vi "Add Terminals to Connector Pane.vi"() -> ()   [LabVIEW 2019]
doc: "Run this VI to assign the controls and indicators of Test - Connector Pane.vi to terminals in the specified connector pane pattern.\n\nFor a list of valid connector pane pattern values, see the Connector Pane Pattern Reference.vi.\n\nThe Detailed Help explains how this example illustrates a general procedure for assigning front panel controls and indicators to a connector pane programmatically."
panel:
  in  "vi path":path=path "Test - Connector Pane.vi"
  in  "Connector Pane Pattern":u32=4814
  # "Select Help>>Show Context Help and move the cursor over the VI icon to display help for this VI.\n\nBefore you start: Open the Detailed Help for this example to display the Configuring a Connector Pane Using VI Scripting topic in the  LabVIEW Help. That topic provides additional details about how this example illustrates the general procedure for assigning front panel controls and indicators to a connector pane programmatically."
  # "Overview: Demonstrates the use of VI Scripting to programmatically assign controls and indicators to a VI's connector pane.\nInstructions:\n1. Open Test - Connector Pane.vi.\n2. Run this VI. Observe the changes to the connector pane of the Test VI."
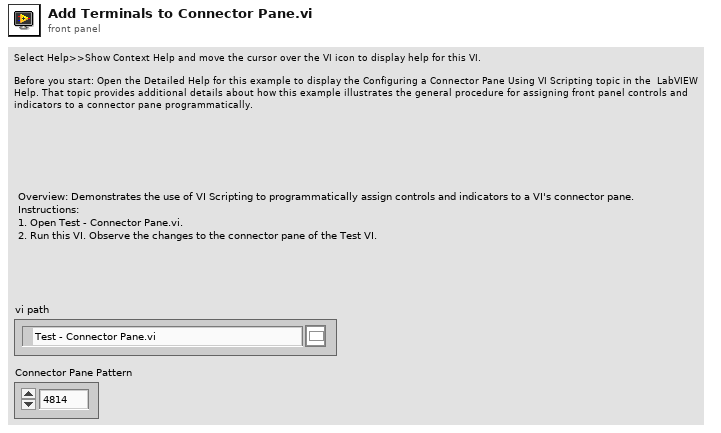
[diagram p1: front panel]
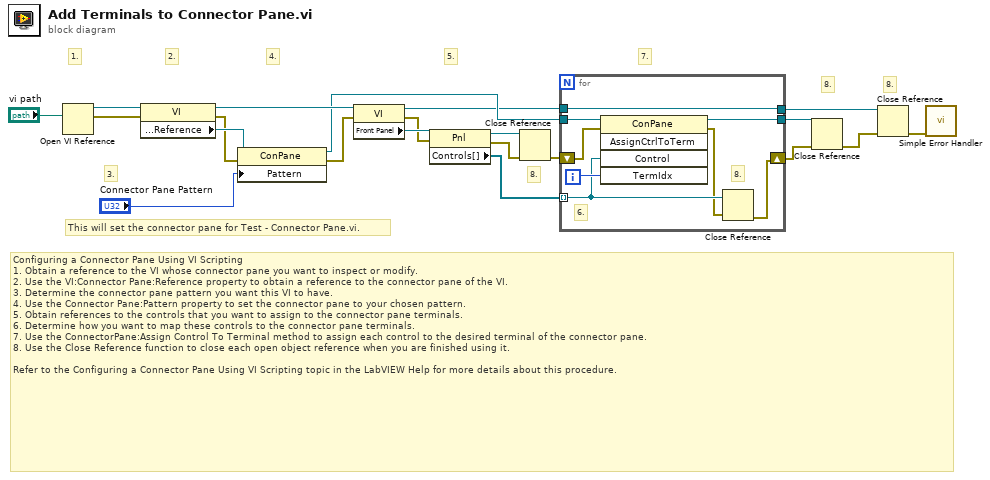
[diagram p0: block diagram]
diagram:
  # "8."
  # "8."
  # "8."
  # "7."
  # "3."
  # "5."
  # "4."
  # "2."
  # "1."
  # "Configuring a Connector Pane Using VI Scripting\n1. Obtain a reference to the VI whose connector pane you want to inspect or modify.\n2. Use the VI:Connector Pane:Reference property to obtain a reference to the connector pane of the VI.\n3. Determine the connector pane pattern you want this VI to have.\n4. Use the Connector Pane:Pattern property to set the connector pane to your chosen pattern.\n5. Obtain references to the controls that you want to assign to the connector pane terminals.\n6. Determine how you want to map these controls to the connector pane terminals.\n7. Use the ConnectorPane:Assign Control To Terminal method to assign each control to the desired terminal of the connector pane.\n8. Use the Close Reference function to close each open object reference when you are finished using it.\n\nRefer to the Configuring a Connector Pane Using VI Scripting topic in the LabVIEW Help for more details about this procedure."
  # "This will set the connector pane for Test - Connector Pane.vi."
  n1 = Open VI Reference(vi path="vi path") -> (vi reference=w2:refnum<vi>, error out=w3:errorcluster)  [unwired: 2 in, 3 out]
  n2 = property class="VI"(reference=w2, error in=w3) -> (reference out=w21:refnum<vi>, error out=w15:errorcluster, "Connector Pane:Reference"=w17:refnum<vi>)
  n3 = property class="ConPane"(reference=w17, error in=w15, "Pattern"="Connector Pane Pattern") -> (reference out=w14:refnum<vi>, error out=w16:errorcluster)
  n4 = property class="VI"(reference=w21, error in=w16) -> (reference out=w13:refnum<vi>, error out=w19:errorcluster, "Front Panel"=w20:refnum<vi>)
  n5 = property class="Pnl"(reference=w20, error in=w19) -> (reference out=w12:refnum<vi>, error out=w11:errorcluster, "Controls[]"=w18:refnum<vi>[])
  n6 = Close Reference(reference=w12, error in (no error)=w11) -> (error out=w10:errorcluster)
  n7 = for {
    tunnel: w18 -> [w24] mode=indexing
    tunnel: w14 -> [w29]
    shift-right: [w25] -> w8
    shift-left: w10 -> [w28]
    tunnel: [w26] -> w6
    tunnel: w13 -> [w26]
    tunnel: [w22] -> w7
    i -> [w27]
    # "8."
    # "6."
    n8 = invoke class="ConPane" method="AssignCtrlToTerm"(reference=w29, error in=w28, "Control"=w24, "TermIdx"=w27) -> (reference out=w22:refnum<vi>, error out=w23:errorcluster)  [unwired: 1 in, 3 out]
    n9 = Close Reference(reference=w24, error in (no error)=w23) -> (error out=w25:errorcluster)
  }
  n10 = Close Reference(reference=w7, error in (no error)=w8) -> (error out=w5:errorcluster)
  n11 = Close Reference(reference=w6, error in (no error)=w5) -> (error out=w1:errorcluster)
  n12 = call <vilib>:"Simple Error Handler.vi"("error in (no error)"=w1) -> ()  [unwired: 4 in, 5 out]
